vi "GUI_Pulsed_wire_scope.vi"() -> ()   [LabVIEW 2013]
uses:
  shared programs/GUI_Template/GUI_master/tcp_new_data_event.ctl
  shared programs/GUI_Template/GUI_master/tcp new data cluster.ctl
panel:
  out "tcp data event":T1
  in  "Refresh Button":bool
  in  "Select device":string(combo)="FrogHPD"
  in  "stop":bool
  out "GUIdevice 1":string="PulsedWireDigitizer"
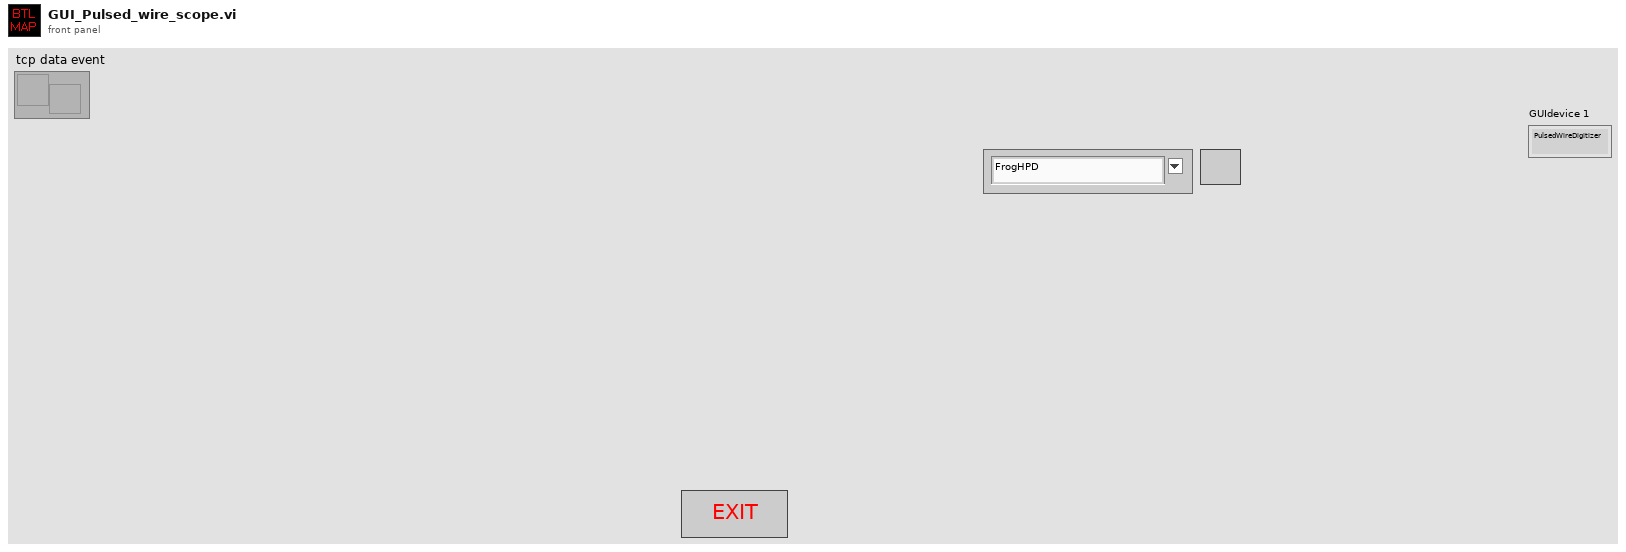
[diagram p1: front panel]
types:
  T1 = typedef "tcp_new_data_event.ctl" = refnum<user-event>
  T2 = enum32{"invalid app kind", "Development System", "Run Time System", "Student Edition", "Embedded LabVIEW", "Evaluation", "Custom"}
  T3 = typedef "tcp new data cluster.ctl" = cluster{"EventEnum":enum16{"new data", "connection status update"}, "Device name":string}
  T4 = enum32{"Invalid", "Standard", "Closed", "Hidden", "Minimized", "Maximized"}
  T5 = cluster{"Core":cluster{"Current VI Reference":refnum<vi>, "Close Panel on Exit?":bool}, "Your Boolean data":bool, "Your string data":string, "SuperGUI":cluster{"STOP queue":refnum<queue>, "SuperGUI ref":refnum<vi>}}
  T6 = cluster{"STOP queue":refnum<queue>, "SuperGUI ref":refnum<vi>}
  T7 = cluster{"Current VI Reference":refnum<vi>, "Close Panel on Exit?":bool}
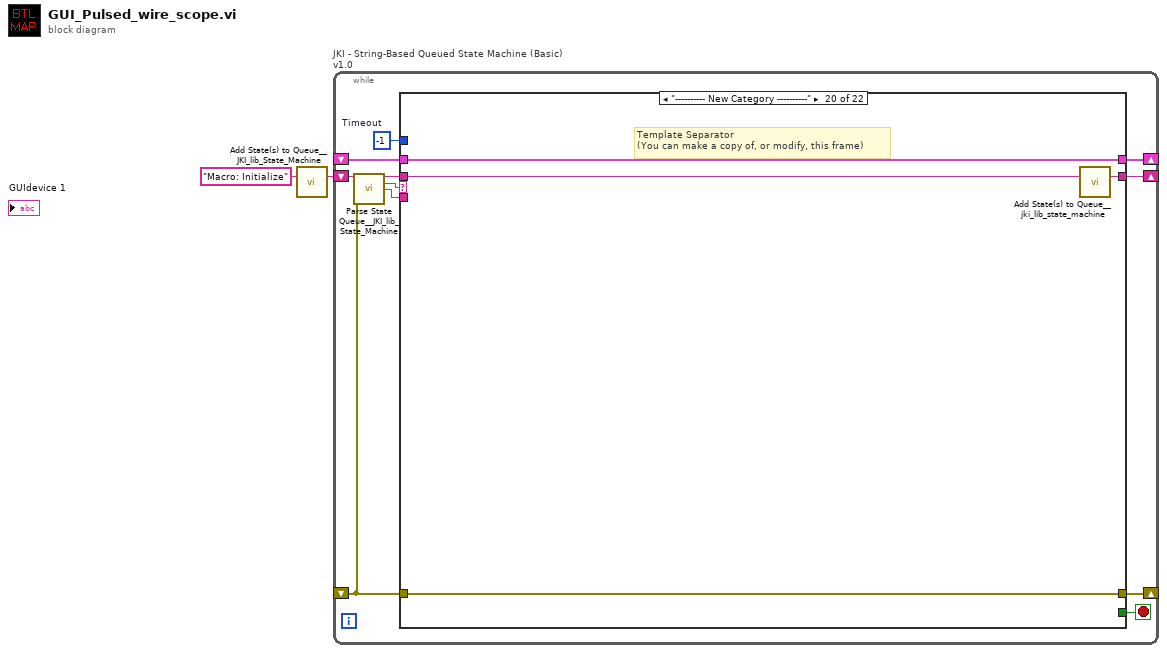
[diagram p0: block diagram]
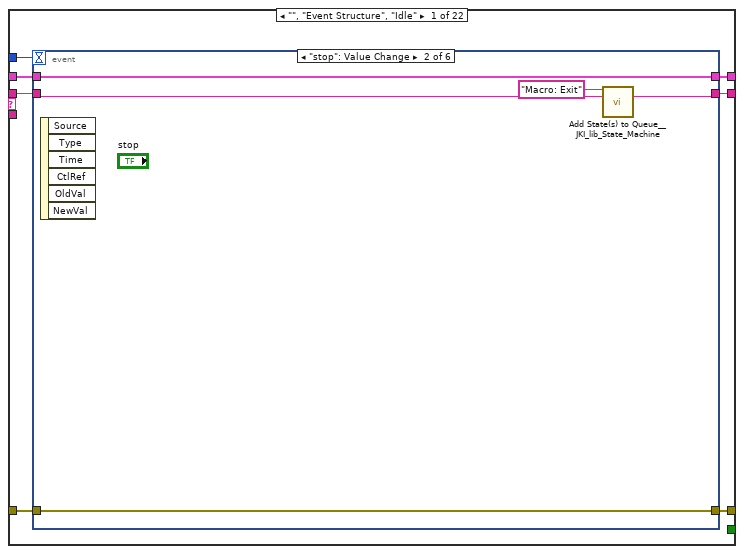
[diagram p2: hidden frame]
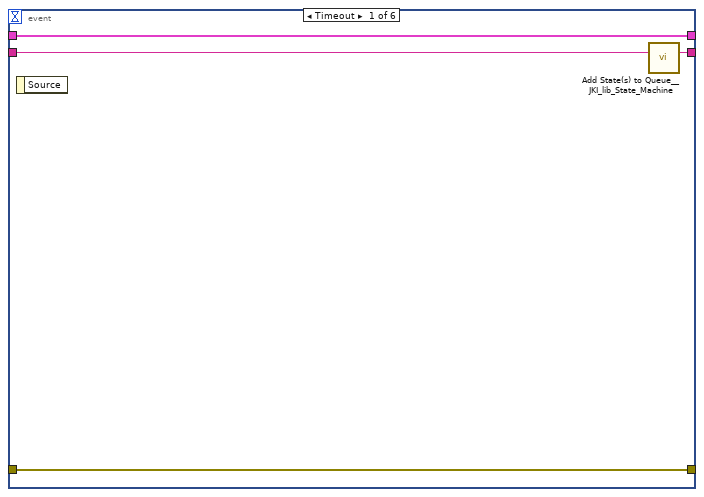
[diagram p3: hidden frame]
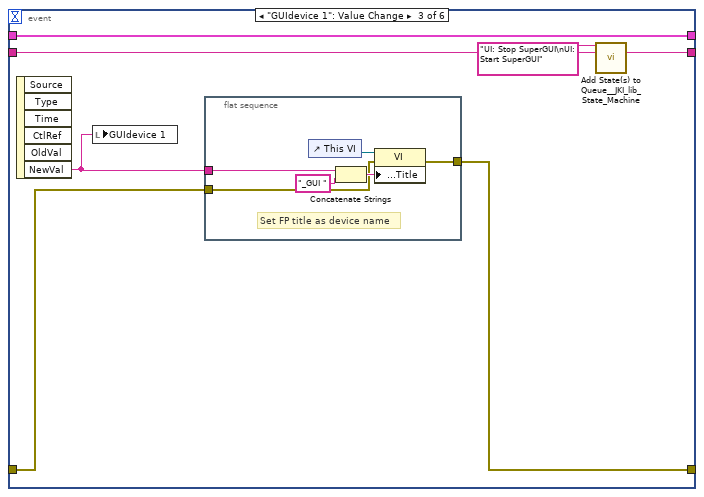
[diagram p4: hidden frame]
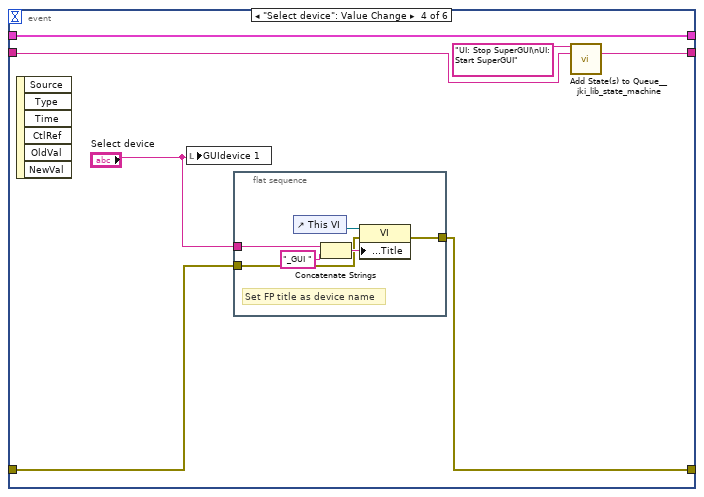
[diagram p5: hidden frame]
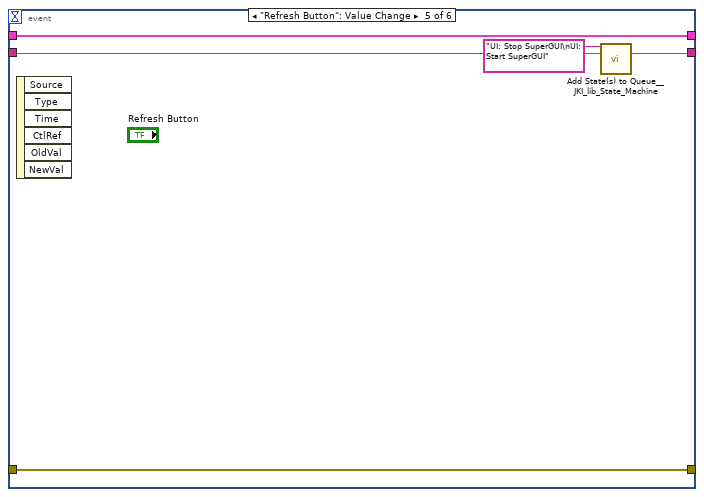
[diagram p6: hidden frame]
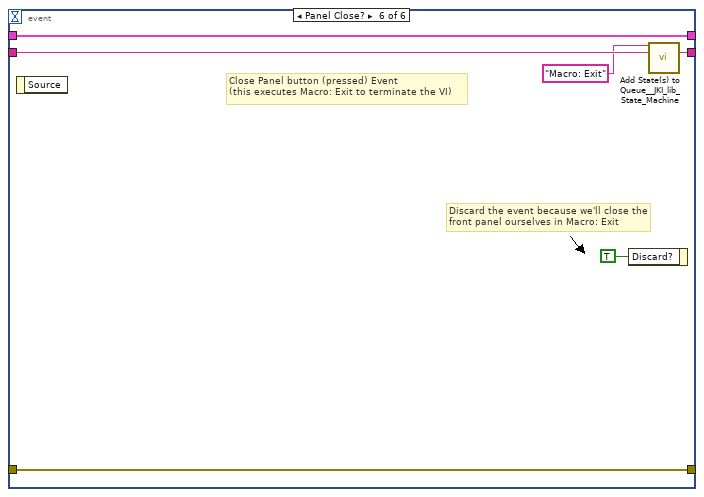
[diagram p7: hidden frame]
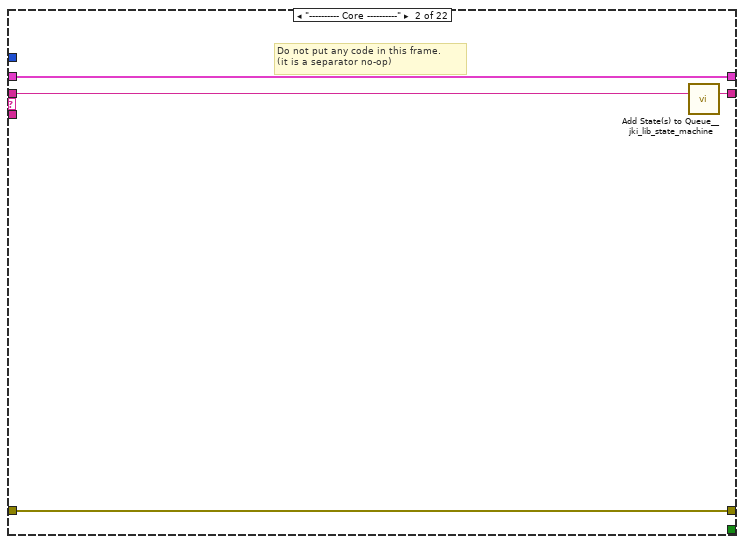
[diagram p8: hidden frame]
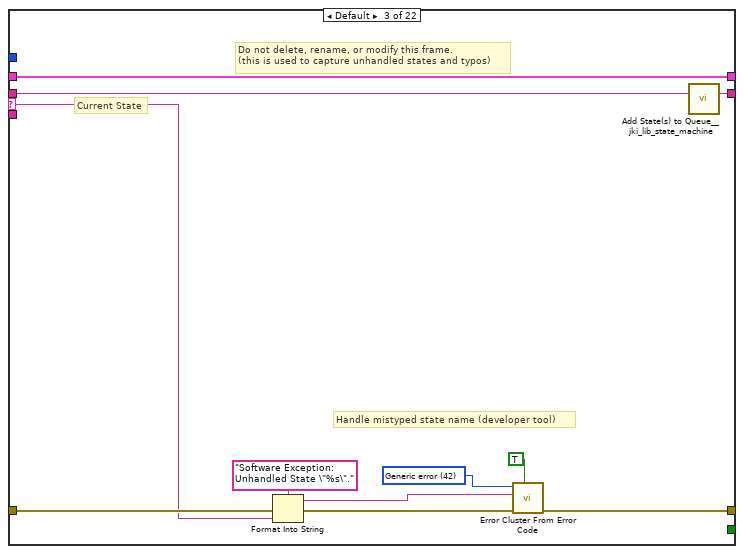
[diagram p9: hidden frame]
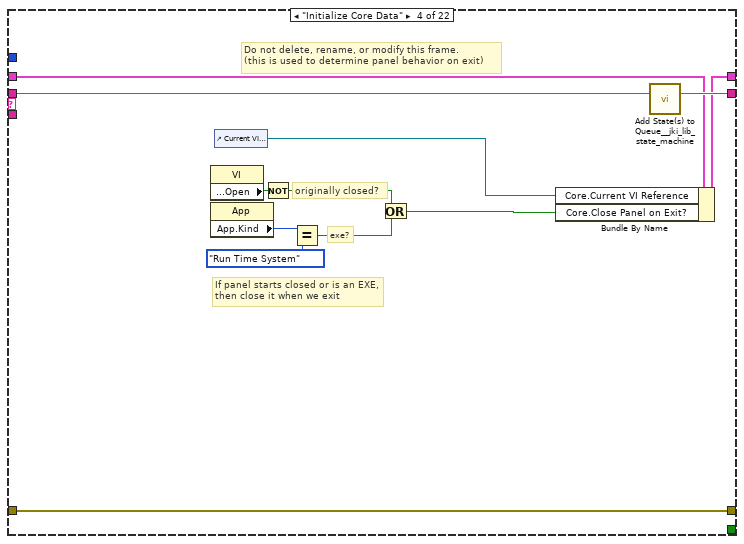
[diagram p10: hidden frame]
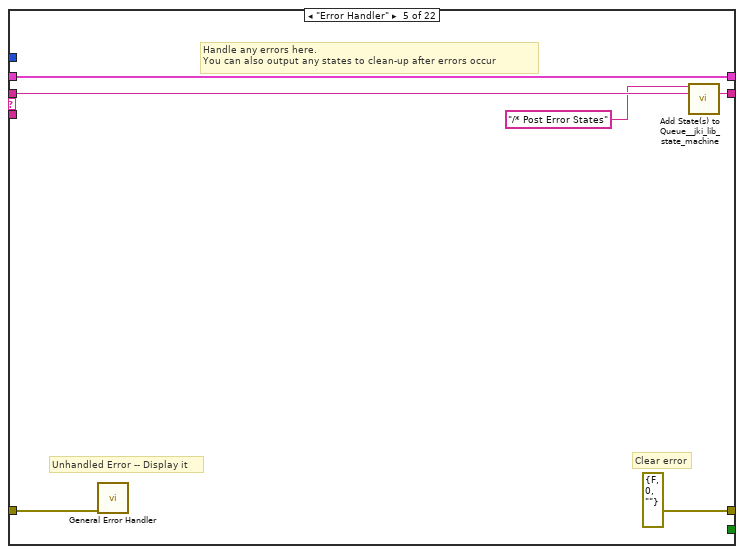
[diagram p11: hidden frame]
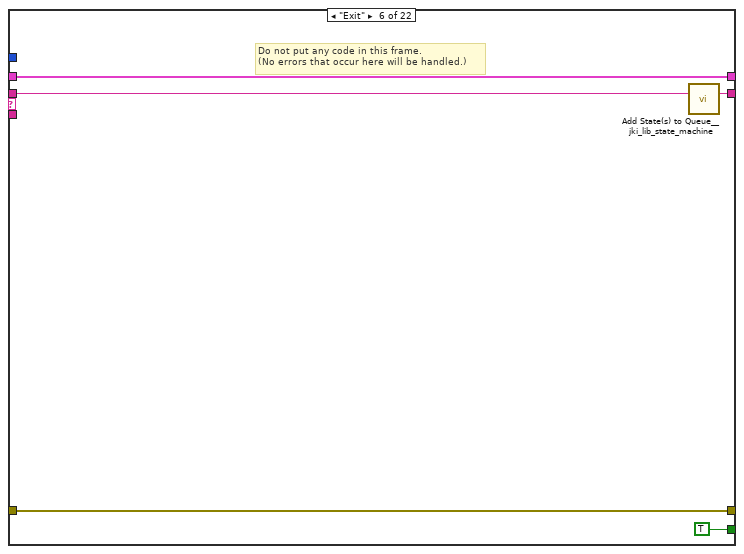
[diagram p12: hidden frame]
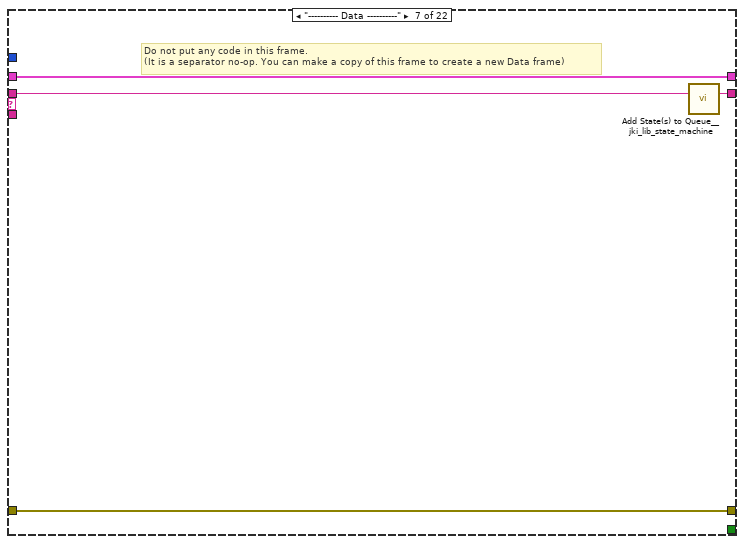
[diagram p13: hidden frame]
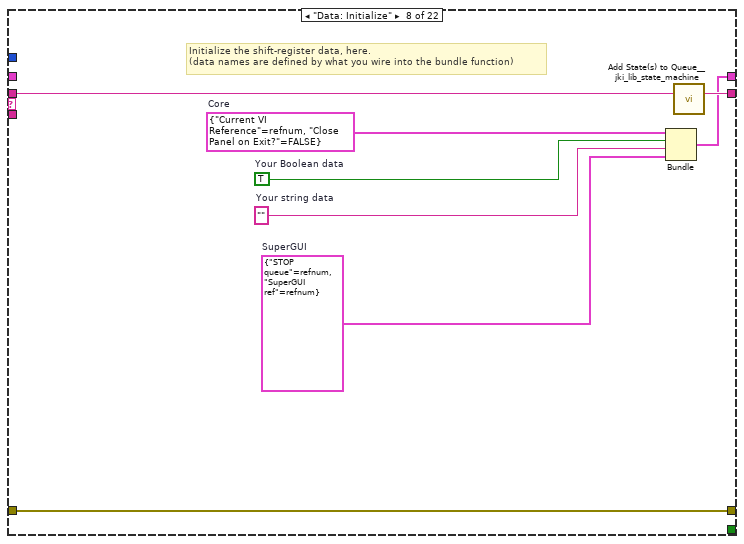
[diagram p14: hidden frame]
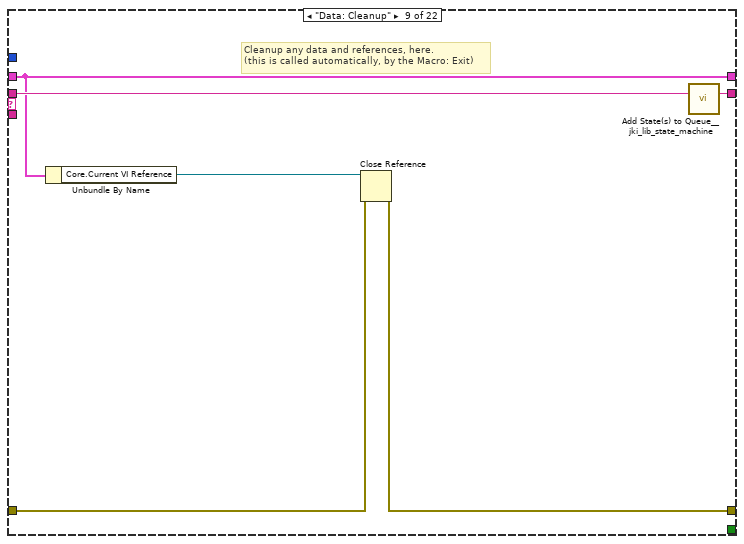
[diagram p15: hidden frame]
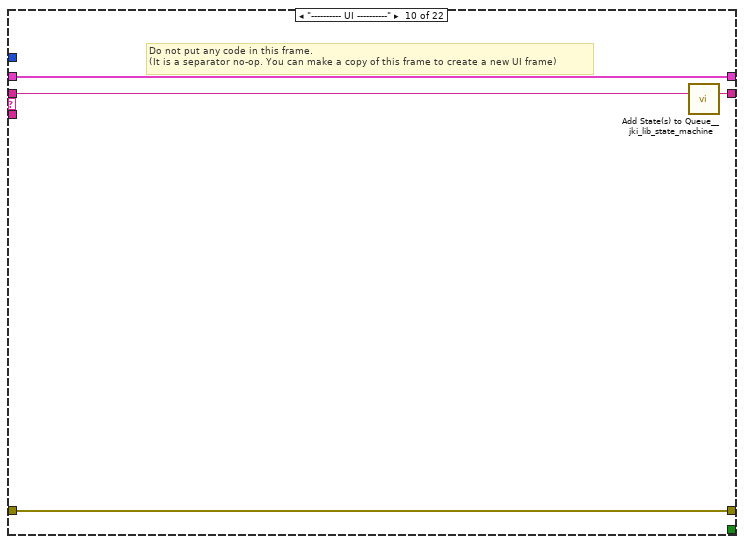
[diagram p16: hidden frame]
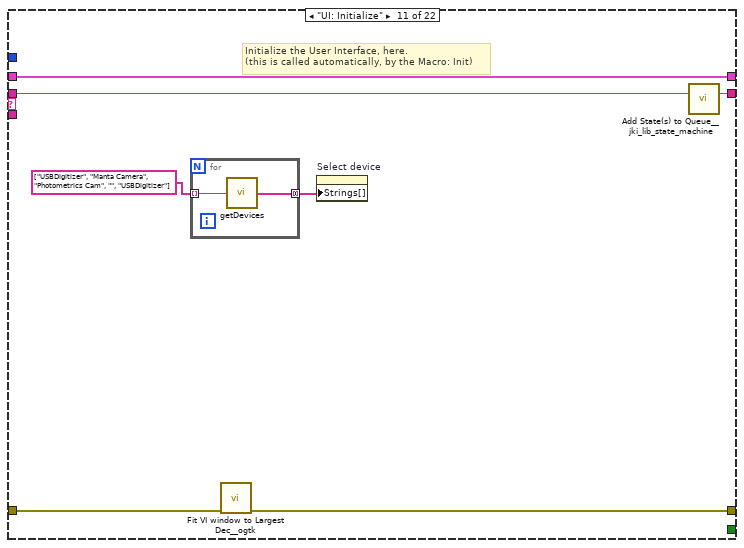
[diagram p17: hidden frame]
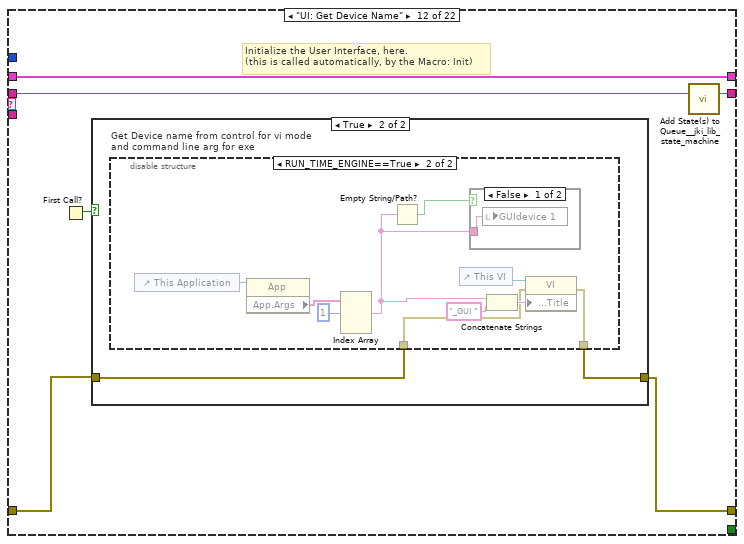
[diagram p18: hidden frame]
diagram:
  n1 = call <vilib>:"Add State(s) to Queue__JKI_lib_State_Machine.vi"("State(s) in (\"\")"="Macro: Initialize") -> ("States Out"=w2:string)  [unwired: 14 in]
  n2 = while "JKI - String-Based Queued State Machine (Basic) v1.0" {
    shift-right: [w6] -> _
    shift-left: _ -> [w5]
    shift-right: [w9] -> _
    shift-left: _ -> [w3]
    shift-right: [w8] -> _
    shift-left: w2 -> [w10]
    stop <- w7 stop-if-true
    w4 = -1  # Timeout
    n3 = call <vilib>:"Parse State Queue__JKI_lib_State_Machine.vi"("State Queue"=w10, "Error In (no error)"=w3) -> ("Remaining States"=w12:string, "Current State"=w13:string, "Arguments"=w11:string)  [unwired: 11 in]
    n4 = case shown="\"---------- New Category ----------\"" w13 {
      selector: w13 -> [_ _ w71 _ _ _ _ _ _ _ _ _ _ _ _ _ _ _ _ _ _ _]
      tunnel: w12 -> [w20 w70 w75 w93 w99 w104 w108 w116 w122 w126 w133 w141 w176 w184 w190 w201 w227 w232 w242 w246 w250 w254]
      tunnel: w11 -> [_ _ _ _ _ _ _ _ _ _ _ _ _ _ w185 w195 _ _ _ _ _ _]
      tunnel: w5 -> [w18 w67 w73 w84 w96 w102 w105 _ w117 w123 w131 w139 w167 w179 w188 w197 w224 w229 w239 w243 w247 w251]
      tunnel: [w17 w68 w77 w90 errorcluster {"status"=FALSE, "code"=0, "source"=""} ("error out") w101 w106 w113 w118 w124 w129 w136 w160 w177 w186 w198 w225 w230 w240 w244 w248 w252] -> w9
      tunnel: w3 -> [w16 w68 w76 w90 w95 w101 w106 w113 w119 w124 w130 w137 w161 w178 w187 w199 w225 w230 w240 w244 w248 w252]
      tunnel: [w19 w69 w74 w92 w98 w103 w107 w115 w121 w125 w132 w140 w175 w183 w189 w200 w226 w231 w241 w245 w249 w253] -> w8
      tunnel: [_ _ _ _ _ TRUE _ _ _ _ _ _ _ _ _ _ _ _ _ _ _ _] -> w7
      tunnel: [w15 w67 w73 w91 w96 w102 w105 w114 w117 w123 w131 w139 w166 w179 w188 w197 w224 w229 w239 w243 w247 w251] -> w6
      tunnel: w4 -> [w14 _ _ _ _ _ _ _ _ _ _ _ _ _ _ _ _ _ _ _ _ _]
      frame "", "Event Structure", "Idle" {
        n5 = event shown="[1] \"stop\": Value Change" {
          selector: _ -> [_ _ _ _ _ _]
          dyn-events: _ -> [_ _ _ _ _ _]
          timeout: w14 -> [_ _ _ _ _ _]
          tunnel: w20 -> [w24 w27 w33 w45 w58 w66]
          tunnel: [w23 w26 w32 w44 w57 w65] -> w19
          tunnel: w18 -> [w21 w29 w36 w49 w60 w63]
          tunnel: [w22 w28 w34 w47 w59 w64] -> w17
          tunnel: w16 -> [w22 w28 w35 w48 w59 w64]
          tunnel: [w21 w29 w36 w49 w60 w63] -> w15
          event Timeout {
            n6 = event-data() -> ()  [unwired: 1 in, 1 out]
            n7 = call <vilib>:"Add State(s) to Queue__JKI_lib_State_Machine.vi"("State(s) in (\"\")"=w24) -> ("States Out"=w23:string)  [unwired: 14 in]
          }
          event "stop": Value Change {
            n8 = event-data() -> ()  [unwired: 1 in, 6 out]
            n9 = call <vilib>:"Add State(s) to Queue__JKI_lib_State_Machine.vi"("State(s) in Front (\"\")"="Macro: Exit", "State(s) in (\"\")"=w27) -> ("States Out"=w26:string)  [unwired: 13 in]
          }
          event "GUIdevice 1": Value Change {
            n10 = event-data() -> ("NewVal"=w30:string)  [unwired: 1 in, 5 out]
            n11 = local write "GUIdevice 1"(w30) -> ()
            n12 = flat-sequence {
              tunnel: [w39] -> w34
              tunnel: w35 -> [w38]
              tunnel: w30 -> [w37]
              frame #0 {
                # "Set FP title as device name"
                n13 = control-ref of="This VI"() -> (w42:refnum<vi>)
                n14 = Concatenate Strings(w37, "_GUI ") -> (w41:string)
                n15 = property class="VI"(reference=w42, error in=w38, "Front Panel.Title"=w41) -> (error out=w39:errorcluster)  [unwired: 1 out]
              }
            }
            n16 = call <vilib>:"Add State(s) to Queue__JKI_lib_State_Machine.vi"("State(s) in Front (\"\")"="UI: Stop SuperGUI\nUI: Start SuperGUI", "State(s) in (\"\")"=w33) -> ("States Out"=w32:string)  [unwired: 13 in]
          }
          event "Select device": Value Change {
            n17 = event-data() -> ()  [unwired: 1 in, 6 out]
            n18 = local write "GUIdevice 1"("Select device") -> ()
            n19 = flat-sequence {
              tunnel: [w52] -> w47
              tunnel: w48 -> [w51]
              tunnel: "Select device" -> [w50]
              frame #0 {
                # "Set FP title as device name"
                n20 = control-ref of="This VI"() -> (w55:refnum<vi>)
                n21 = Concatenate Strings(w50, "_GUI ") -> (w54:string)
                n22 = property class="VI"(reference=w55, error in=w51, "Front Panel.Title"=w54) -> (error out=w52:errorcluster)  [unwired: 1 out]
              }
            }
            n23 = call <vilib>:"Add State(s) to Queue__jki_lib_state_machine.vi"("State(s) in Front (\"\")"="UI: Stop SuperGUI\nUI: Start SuperGUI", "State(s) in (\"\")"=w45) -> ("States Out"=w44:string)  [unwired: 13 in]
          }
          event "Refresh Button": Value Change {
            n24 = event-data() -> ()  [unwired: 1 in, 6 out]
            n25 = call <vilib>:"Add State(s) to Queue__JKI_lib_State_Machine.vi"("State(s) in Front (\"\")"="UI: Stop SuperGUI\nUI: Start SuperGUI", "State(s) in (\"\")"=w58) -> ("States Out"=w57:string)  [unwired: 13 in]
          }
          event Panel Close? {
            # "Discard the event because we'll close the front panel ourselves in Macro: Exit"
            # "Close Panel button (pressed) Event\n(this executes Macro: Exit to terminate the VI)"
            n26 = event-data() -> ()  [unwired: 1 in, 1 out]
            n27 = event-data("Discard?"=TRUE) -> ()  [unwired: 1 in, 1 out]
            n28 = call <vilib>:"Add State(s) to Queue__JKI_lib_State_Machine.vi"("State(s) in Front (\"\")"="Macro: Exit", "State(s) in (\"\")"=w66) -> ("States Out"=w65:string)  [unwired: 13 in]
          }
        }
      }
      frame "---------- Core ----------" {
        # "Do not put any code in this frame.\n(it is a separator no-op)"
        n29 = call <vilib>:"Add State(s) to Queue__jki_lib_state_machine.vi"("State(s) in (\"\")"=w70) -> ("States Out"=w69:string)  [unwired: 14 in]
      }
      frame Default {
        w80 = 42 items=["No error", "Argument error", "Memory is full", "Out of zone", "End of file", "File already open", "Generic file I/O error", "File not found", "File permission error", "Disk is full", "Duplicate path", "Too many files open", "System feature not enabled", "Resource file not found", "Cannot add resource", "Resource not found", "Image not found", "Image memory error", "Pen does not exist", "Config type invalid", "Config token not found", "Config parse error", "Config memory error", "Bad external code format", "Bad external code offset", "External code not present", "Null window", "Destroy window error", "Null menu", "Print aborted", "Bad print record", "Print driver error", "Windows error during printing", "Memory error during printing", "Print dialog error", "Generic print error", "Invalid device refnum", "Device not found", "Device parameter error", "Device unit error", "Cannot open device", "Device call aborted", "Generic error", "Cancelled by user", "Object ID too low", "Object ID too high", "Object not in heap", "Unknown heap", "Unknown object (invalid DefProc)", "Unknown object (DefProc not in table)", "Message out of range", "Invalid (null) method", "Unknown message", "Manager call not supported", "Bad address", "Network operation in progress", "Network operation timed out", "Connection is busy", "Network attribute not supported", "Network error", "Address in use", "System out of memory", "Connection aborted", "Connection refused", "Not connected", "Already connected", "Connection closed", "Initialization error (interapplication manager)", "Bad occurrence", "Wait on unbound occurrence handler", "Occurrence queue overflow", "Datalog type conflict", "Unused", "Unrecognized type (interapplication manager)", "Memory corrupt", "Failed to make temporary DLL", "Old CIN version", "Drag socket not found", "Failed to load drop-object", "Failed to register OLE object", "Failed to release OLE object", "Format specifier type mismatch", "Unknown format specifier", "Too few format specifiers", "Too many format specifiers", "Scan failed", "Newer CIN version", "Error converting to variant", "Runtime menu error", "Password tampered", "Variant attribute not found", "Incompatible variant data type", "Event data is not available", "Event Store is not present", "Occurrence is not found", "Event Queue is not created", "Event info is not available", "Refnum passed is NULL", "Error retrieving Class GUID", "Error retrieving CoClass GUID", "Error retrieving TypeLib GUID.", "Bad built application magic bytes.", "Specific driver is different from the specific driver associated with the Logical Name.", "There is no session opened to the class driver.", "Max Error", "MAX - Error with config objects", "MAX - Error loading configuration", "MAX - Group not supported"]
        # "Current State"
        # "Do not delete, rename, or modify this frame.\n(this is used to capture unhandled states and typos)"
        # "Handle mistyped state name (developer tool)"
        n30 = Format Into String(format string="Software Exception: Unhandled State \"%s\"." ("message"), error in=w76, w71) -> (resulting string=w79:string, error out=w78:errorcluster)  [unwired: 1 in]
        n31 = call <vilib>:"Error Cluster From Error Code.vi"("show call chain? (False)"=TRUE, "error in (no error)"=w78, "error message (\"\")"=w79, "error code (0)"=w80) -> ("error out"=w77:errorcluster)  [unwired: 5 in]
        n32 = call <vilib>:"Add State(s) to Queue__jki_lib_state_machine.vi"("State(s) in (\"\")"=w75) -> ("States Out"=w74:string)  [unwired: 14 in]
      }
      frame "Initialize Core Data" {
        # "Do not delete, rename, or modify this frame.\n(this is used to determine panel behavior on exit)"
        # "originally closed?"
        # "exe?"
        # "If panel starts closed or is an EXE, then close it when we exit"
        n33 = property class="VI"() -> ("Front Panel.Open"=w89:bool)  [unwired: 2 in, 2 out]
        n34 = property class="App"() -> ("App.Kind"=w88:T2)  [unwired: 2 in, 2 out]
        n35 = control-ref of="Current VI Reference"() -> (w82:refnum<vi>)
        n36 = Not(x=w89) -> (.not. x?=w86:bool)
        n37 = Equal?(x=w88, y=T2."Run Time System" ("Application:Kind")) -> (x = y?=w85:bool)
        n38 = Or(x=w86, y=w85) -> (x .or. y?=w83:bool)
        n39 = Bundle By Name(cluster=w84, "Core.Current VI Reference"=w82, "Core.Close Panel on Exit?"=w83) -> (w91:T5)
        n40 = call <vilib>:"Add State(s) to Queue__jki_lib_state_machine.vi"("State(s) in (\"\")"=w93) -> ("States Out"=w92:string)  [unwired: 14 in]
      }
      frame "Error Handler" {
        # "Unhandled Error -- Display it"
        # "Handle any errors here.\nYou can also output any states to clean-up after errors occur"
        # "Clear error"
        n41 = call <vilib>:"General Error Handler.vi"("error in (no error)"=w95) -> ()  [unwired: 10 in, 5 out]
        n42 = call <vilib>:"Add State(s) to Queue__jki_lib_state_machine.vi"("State(s) in Front (\"\")"="/* Post Error States", "State(s) in (\"\")"=w99) -> ("States Out"=w98:string)  [unwired: 13 in]
      }
      frame "Exit" {
        # "Do not put any code in this frame.\n(No errors that occur here will be handled.)"
        n43 = call <vilib>:"Add State(s) to Queue__jki_lib_state_machine.vi"("State(s) in (\"\")"=w104) -> ("States Out"=w103:string)  [unwired: 14 in]
      }
      frame "---------- Data ----------" {
        # "Do not put any code in this frame.\n(It is a separator no-op. You can make a copy of this frame to create a new Data frame)"
        n44 = call <vilib>:"Add State(s) to Queue__jki_lib_state_machine.vi"("State(s) in (\"\")"=w108) -> ("States Out"=w107:string)  [unwired: 14 in]
      }
      frame "Data: Initialize" {
        w109 = T6 {"STOP queue"=refnum, "SuperGUI ref"=refnum}  # SuperGUI
        w110 = T7 {"Current VI Reference"=refnum, "Close Panel on Exit?"=FALSE}  # Core
        w112 = TRUE  # Your Boolean data
        w111 = ""  # Your string data
        # "Initialize the shift-register data, here.\n(data names are defined by what you wire into the bundle function)"
        n45 = Bundle("Core"=w110, "Your Boolean data"=w112, "Your string data"=w111, "SuperGUI"=w109) -> (w114:T5)  [unwired: 1 in]
        n46 = call <vilib>:"Add State(s) to Queue__jki_lib_state_machine.vi"("State(s) in (\"\")"=w116) -> ("States Out"=w115:string)  [unwired: 14 in]
      }
      frame "Data: Cleanup" {
        # "Cleanup any data and references, here.\n(this is called automatically, by the Macro: Exit)"
        n47 = Unbundle By Name(w117) -> ("Core.Current VI Reference"=w120:refnum<vi>)
        n48 = Close Reference(reference=w120, error in (no error)=w119) -> (error out=w118:errorcluster)
        n49 = call <vilib>:"Add State(s) to Queue__jki_lib_state_machine.vi"("State(s) in (\"\")"=w122) -> ("States Out"=w121:string)  [unwired: 14 in]
      }
      frame "---------- UI ----------" {
        # "Do not put any code in this frame.\n(It is a separator no-op. You can make a copy of this frame to create a new UI frame)"
        n50 = call <vilib>:"Add State(s) to Queue__jki_lib_state_machine.vi"("State(s) in (\"\")"=w126) -> ("States Out"=w125:string)  [unwired: 14 in]
      }
      frame "UI: Initialize" {
        # "Initialize the User Interface, here.\n(this is called automatically, by the Macro: Init)"
        n51 = for {
          tunnel: string[] ["USBDigitizer", "Manta Camera", "Photometrics Cam", "", "USBDigitizer"] -> [w135] mode=indexing
          tunnel: [w134] -> w127 mode=concatenating
          n52 = call "getDevices.vi"("Device Class"=w135) -> ("All Devices"=w134:string[])
        }
        n53 = call <userlib>:"Fit VI window to Largest Dec__ogtk.vi"("error in (no error)"=w130) -> ("error out"=w129:errorcluster)  [unwired: 5 in, 1 out]
        n54 = property on="Select device" class="CmbBox"("Strings[]"=w127) -> ()  [unwired: 2 in, 2 out]
        n55 = call <vilib>:"Add State(s) to Queue__jki_lib_state_machine.vi"("State(s) in (\"\")"=w133) -> ("States Out"=w132:string)  [unwired: 14 in]
      }
      frame "UI: Get Device Name" {
        # "Initialize the User Interface, here.\n(this is called automatically, by the Macro: Init)"
        n56 = First Call?() -> (First Call?: T/F=w138:bool)
        n57 = case shown="True" w138 {
          tunnel: w137 -> [w142 w144]
          tunnel: [w142 w143] -> w136
          frame False {
          }
          frame True {
            n58 = disable-structure "Get Device name from control for vi mode\nand command line arg for exe" shown="RUN_TIME_ENGINE==True" {
              disable-tunnel: w144 -> [w145 w147]
              disable-tunnel: [w145 w146] -> w143
              frame condition #0 (active) {
              }
              frame condition #1 {
                n59 = control-ref of="This Application"() -> (w155:refnum<vi>)
                n60 = property class="App"(reference=w155) -> ("App.Args"=w154:string[])  [unwired: 1 in, 2 out]
                n61 = Index Array(array=w154, index #1=1 ("index")) -> (element #1=w148:string)  [unwired: 2 in, 2 out]
                n62 = Empty String/Path?(string/path=w148) -> (empty?=w152:bool)
                n63 = control-ref of="This VI"() -> (w151:refnum<vi>)
                n64 = case shown="False" w152 {
                  tunnel: w148 -> [w156 _]
                  frame False {
                    n65 = local write "GUIdevice 1"(w156) -> ()
                  }
                  frame True {
                  }
                }
                n66 = Concatenate Strings(w148, "_GUI ") -> (w150:string)
                n67 = property class="VI"(reference=w151, error in=w147, "Front Panel.Title"=w150) -> (error out=w146:errorcluster)  [unwired: 1 out]
              }
            }
          }
        }
        n68 = call <vilib>:"Add State(s) to Queue__jki_lib_state_machine.vi"("State(s) in (\"\")"=w141) -> ("States Out"=w140:string)  [unwired: 14 in]
      }
      frame "UI: Start SuperGUI" {
        # "create stop queue for supergui and its clones"
        # "x100 abort will be dependent on caller VI\nx80 abort will be independent of caller vi, this will abort vi when labview is closed."
        # "Start SuperGUI asynchronous way"
        n69 = vi-ref "GUI_Master_subvi_reentrant_queues.vi"() -> (w159:refnum<vi>)
        n70 = property class="VI"(reference=w159) -> ("Path"=w158:path)  [unwired: 1 in, 2 out]
        n71 = Create User Event(user event datatype=T3 {"EventEnum"=enum."new data", "Device name"="Device name"} ("New Event"), error in=w161) -> (user event=w162:refnum<user-event>, error out=w168:errorcluster)
        "tcp data event" <- w162
        n72 = control-ref of="This Application"() -> (w165:refnum<vi>)
        n73 = control-ref of="This VI"() -> (w164:refnum<vi>)
        n74 = Open VI Reference(type specifier VI Refnum (for type only)=refnum<vi> refnum, vi path=w158, options=256) -> (vi reference=w174:refnum<vi>, error out=w173:errorcluster)  [unwired: 3 in]
        n75 = register-events(w162) -> ()  [unwired: 2 in, 2 out]
        n76 = call "supergui create stop queue.vi"() -> ("STOP Queue out"=w170:refnum<queue>)  [unwired: 11 in]
        n77 = Current VI's Menubar() -> (w163:refnum<k9>)
        n78 = call-by-ref "Start Asynchronous Call"(reference=w174, error in=w173, "STOP Queue in"=w170, "This Application"=w165, 8:"error in (no error)"=w168, "tcp data event"=w162, "Caller menu reference"=w163, "Caller VI ref"=w164) -> (reference out=w157:refnum<vi>, error out=w160:errorcluster)  [unwired: 5 in, 1 out]
        n79 = Bundle By Name(cluster=w167, "SuperGUI.SuperGUI ref"=w157, "SuperGUI.STOP queue"=w170) -> (w166:T5)
        n80 = call <vilib>:"Add State(s) to Queue__jki_lib_state_machine.vi"("State(s) in (\"\")"=w176) -> ("States Out"=w175:string)  [unwired: 14 in]
      }
      frame "UI: Stop SuperGUI" {
        # "Stop Supergui Clone and wait until it exit properly"
        n81 = Unbundle By Name(w179) -> ("SuperGUI.SuperGUI ref"=w181:refnum<vi>, "SuperGUI.STOP queue"=w180:refnum<queue>)
        n82 = Release Queue(queue=w180, error in (no error)=w178) -> (error out=w182:errorcluster)  [unwired: 1 in, 2 out]
        n83 = call-by-ref "Wait On Asynchronous Call"(reference=w181, error in=w182) -> ("error out"=w177:errorcluster)  [unwired: 11 in, 2 out]
        n84 = call <vilib>:"Add State(s) to Queue__jki_lib_state_machine.vi"("State(s) in (\"\")"=w184) -> ("States Out"=w183:string)  [unwired: 14 in]
      }
      frame "UI: Cursor Set" {
        # "Argument"
        # "Set and Unset Cursor Busy.\n(Usage: \"UI: Cursor Set >> Busy|Idle\")"
        n85 = case shown="\"Idle\", Default" w185 {
          tunnel: w187 -> [w192 w194]
          tunnel: [w191 w193] -> w186
          frame "Idle", Default {
            n86 = call <vilib>:"Unset Busy.vi"("error in (no error)"=w192) -> ("error out"=w191:errorcluster)  [unwired: 10 in]
          }
          frame "Busy" {
            n87 = call <vilib>:"Set Busy.vi"("error in (no error)"=w194) -> ("error out"=w193:errorcluster)  [unwired: 9 in, 1 out]
          }
        }
        n88 = call <vilib>:"Add State(s) to Queue__jki_lib_state_machine.vi"("State(s) in (\"\")"=w190) -> ("States Out"=w189:string)  [unwired: 14 in]
      }
      frame "UI: Front Panel State" {
        # "Argument"
        # "Set Front Panel Open or Closed\n(Usage: \"UI: Front Panel State >> Open|Close\")"
        n89 = Unbundle By Name(w197) -> ("Core.Current VI Reference"=w196:refnum<vi>)
        n90 = case shown="\"Open\", Default" w195 {
          tunnel: w199 -> [w205 w218]
          tunnel: [w207 w219] -> w198
          tunnel: w196 -> [w206 w216]
          frame "Open", Default {
            n91 = property class="VI"(reference=w206, error in=w205) -> (reference out=w203:refnum<vi>, error out=w204:errorcluster, "Front Panel.Open"=w202:bool)
            n92 = case shown="False" w202 {
              tunnel: [w210 w213] -> w207
              tunnel: w204 -> [w209 w213]
              tunnel: w203 -> [w208 _]
              frame False {
                n93 = invoke class="VI" method="FP.Open"(reference=w208, error in=w209, "Activate"=TRUE, "State"=T4."Standard") -> (error out=w210:errorcluster)  [unwired: 1 in, 4 out]
              }
              frame True {
              }
            }
          }
          frame "Close" {
            n94 = property class="VI"(reference=w216, error in=w218) -> (reference out=w215:refnum<vi>, error out=w217:errorcluster, "Front Panel.Open"=w214:bool)
            n95 = case shown="True" w214 {
              tunnel: [w220 w223] -> w219
              tunnel: w217 -> [w220 w222]
              tunnel: w215 -> [_ w221]
              frame False {
              }
              frame True {
                n96 = invoke class="VI" method="FP.Close"(reference=w221, error in=w222) -> (error out=w223:errorcluster)  [unwired: 1 in, 2 out]
              }
            }
          }
        }
        n97 = call <vilib>:"Add State(s) to Queue__jki_lib_state_machine.vi"("State(s) in (\"\")"=w201) -> ("States Out"=w200:string)  [unwired: 14 in]
      }
      frame "---------- Macro ----------" {
        # "Do not put any code in this frame.\n(It is a separator no-op. You can make a copy of this frame to create a new Macro frame)"
        n98 = call <vilib>:"Add State(s) to Queue__jki_lib_state_machine.vi"("State(s) in (\"\")"=w227) -> ("States Out"=w226:string)  [unwired: 14 in]
      }
      frame "Macro: Initialize" {
        # "Initialization Macro\n(This is called once, when the VI starts)"
        n99 = call <vilib>:"Add State(s) to Queue__jki_lib_state_machine.vi"("State(s) in Front (\"\")"="Data: Initialize\nInitialize Core Data\nUI: Initialize\nUI: Get Device Name\nUI: Start SuperGUI\nUI: Front Panel State >> Open", "State(s) in (\"\")"=w232) -> ("States Out"=w231:string)  [unwired: 13 in]
      }
      frame "Macro: Exit" {
        # "Exit Macro\n(This is called once, when the VI exits)"
        n100 = Unbundle By Name(w239) -> ("Core.Close Panel on Exit?"=w238:bool)
        n101 = Select(t="UI: Front Panel State >> Close", s=w238, f="") -> (s? t:f=w235:string)
        n102 = call <vilib>:"Add State(s) to Queue__jki_lib_state_machine.vi"("State(s) in (\"\")"=w235, "State(s) at Back (\"\")"="Data: Cleanup\nExit") -> ("States Out"=w233:string)  [unwired: 13 in]
        n103 = call <vilib>:"Add State(s) to Queue__jki_lib_state_machine.vi"("State(s) in Front (\"\")"=w233, "State(s) in (\"\")"=w242) -> ("States Out"=w241:string)  [unwired: 13 in]
      }
      frame "---------- New Category ----------" {
        # "Template Separator\n(You can make a copy of, or modify, this frame)"
        n104 = call <vilib>:"Add State(s) to Queue__jki_lib_state_machine.vi"("State(s) in (\"\")"=w246) -> ("States Out"=w245:string)  [unwired: 14 in]
      }
      frame "New Category: 1" {
        # "Your code here.\n(You can make a copy of, or modify, this frame)"
        n105 = call <vilib>:"Add State(s) to Queue__jki_lib_state_machine.vi"("State(s) in (\"\")"=w250) -> ("States Out"=w249:string)  [unwired: 14 in]
      }
      frame "New Category: 2" {
        # "Your code here.\n(You can make a copy of, or modify, this frame)"
        n106 = call <vilib>:"Add State(s) to Queue__jki_lib_state_machine.vi"("State(s) in (\"\")"=w254) -> ("States Out"=w253:string)  [unwired: 14 in]
      }
    }
  }
